vi "WFPadToEvenSamplesA.vi"(4 "error in (no error)":errorcluster, 6 "Baseline":dbl, 7 "Waveform In":waveform(dbl)={"t0"=timestamp(0 s since 1904-01-01), "dt"=0.0, "Y"=[]}) -> (0 "error out":errorcluster, 3 "Waveform Out":waveform(dbl))   [LabVIEW 2013]
uses:
  <vilib>/Waveform/WDTOps.llb/WDT Number of Waveform Samples DBL.vi
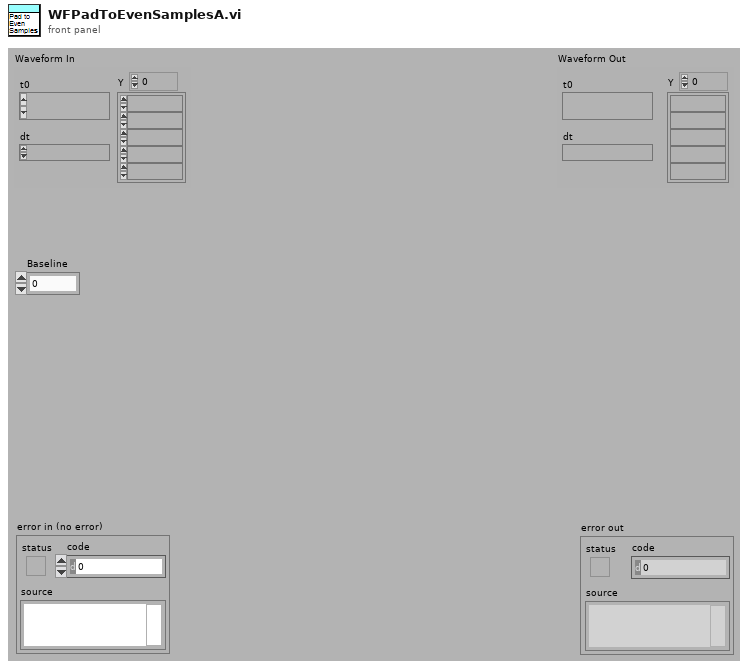
[diagram p1: front panel]
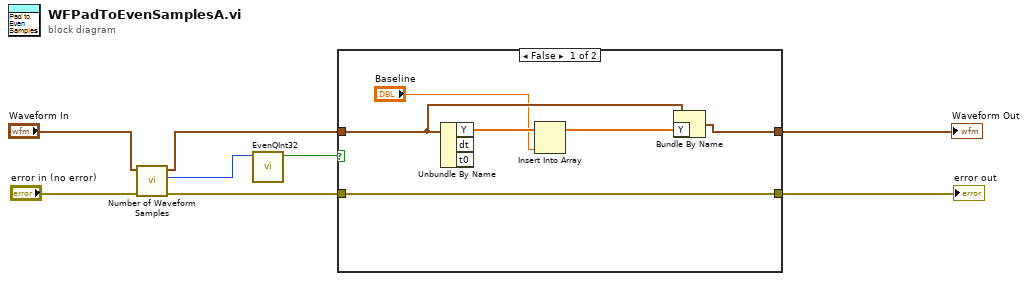
[diagram p0: block diagram]
diagram:
  n1 = call-poly <vilib>:"Number of Waveform Samples.vi"("error in (no error)"="error in (no error)", "waveform in"="Waveform In") -> ("error out"=w7:errorcluster, "number of samples"=w4:i32, "waveform out"=w3:waveform(dbl))  [unwired: 7 in]
  n2 = call "EvenQInt32.vi"("Input"=w4) -> ("Result"=w2:bool)  [unwired: 10 in]
  n3 = case shown="False" w2 {
    tunnel: w7 -> [w12 w16]
    tunnel: [w12 w16] -> w6
    tunnel: w3 -> [w10 w15]
    tunnel: [w13 w15] -> w1
    frame False {
      n4 = Unbundle By Name(w10) -> ("Y"=w14:dbl[])  [unwired: 2 out]
      n5 = Insert Into Array(array=w14, new element="Baseline") -> (w11:dbl[])  [unwired: 1 in]
      n6 = Bundle By Name(cluster=w10, "Y"=w11) -> (w13:waveform(dbl))
    }
    frame True {
    }
  }
  "Waveform Out" <- w1
  "error out" <- w6
